vi "2400_4probesweep.vi"() -> ()   [LabVIEW 2021]
doc: "Configures a sweep and takes voltage and current readings at each point."
uses:
  <instrlib>/Keithley 24XX/Public/Data/Read (Multiple Points).vi
  <instrlib>/Keithley 24XX/Keithley 24XX.lvlib
  <vilib>/Analysis/NI_AALPro.lvlib
panel:
  out "Resistivity":dbl
  in  "Correction factor":dbl
  out "error out":errorcluster
  out "Intercept":dbl
  out "Slope":dbl
  out "XY Graph":cluster{"Current":sgl[], "Array":dbl[]}[](graph)
  in  "Source Mode  (0: Voltage)":u16(ring) items=["Voltage", "Current"]
  in  "Serial Configuration":T1={"Baud Rate"=9600, "Parity"=0, "Data Bits"=8, "Stop Bits"=10, "Flow Control"=0} {"Flow Control" items=["None", "XON/XOFF", "RTS/CTS", "XON/XOFF & RTS/CTS", "DTR/DSR", "XON/XOFF & DTR/DSR"]; "Stop Bits" items=["1.0"=10, "1.5"=15, "2.0"=20]; "Data Bits" items=["7"=7, "8"=8]; "Parity" items=["None", "Odd", "Even", "Mark", "Space"]; "Baud Rate" items=["300"=300, "600"=600, "1200"=1200, "2400"=2400, "4800"=4800, "9600"=9600, "19200"=19200]}
  in  "VISA resource name":refnum<visa-resource-name>
  out "Waveform Graph":sgl[][](graph)
  in  "Timeout (10000 ms)":i32=10000 format="%#.6g"
  in  "Maximum Amplitude (2)":dbl=2.0
  in  "Minimum Amplitude (1)":dbl=1.0
  in  "Number of Points (5)":u32=5
  in  "Compliance  Level (0.1)":dbl=0.1
  # "(c) 2006 - 2015 National Instruments.  ALL RIGHTS RESERVED."
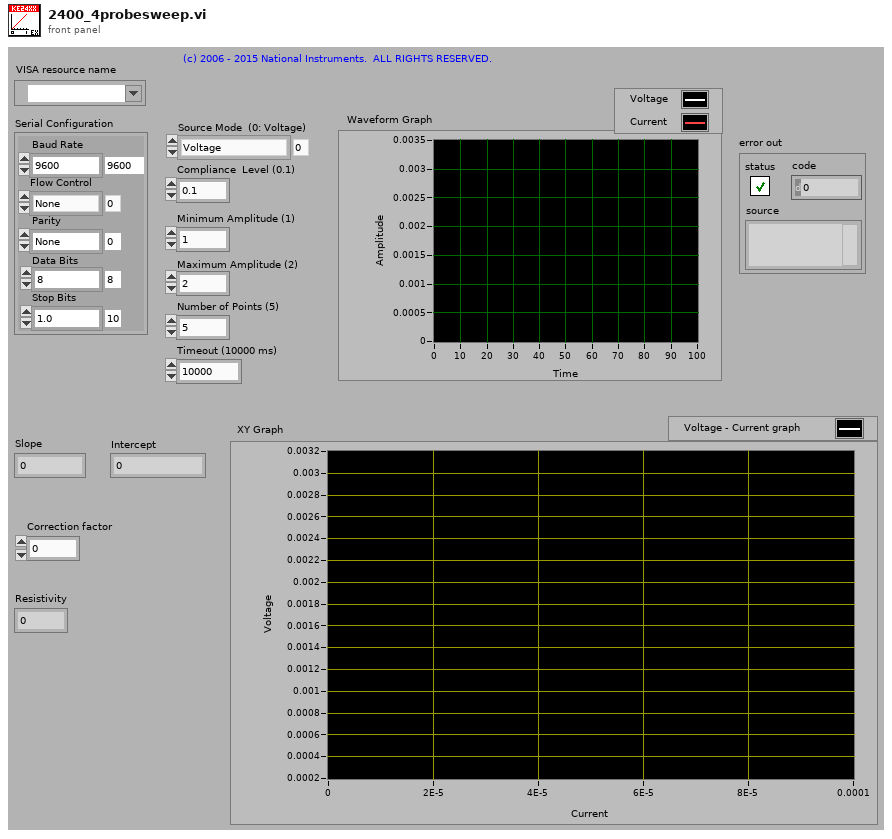
[diagram p1: front panel]
types:
  T1 = cluster{"Baud Rate":u32, "Parity":u16, "Data Bits":u16, "Stop Bits":u16, "Flow Control":u16}
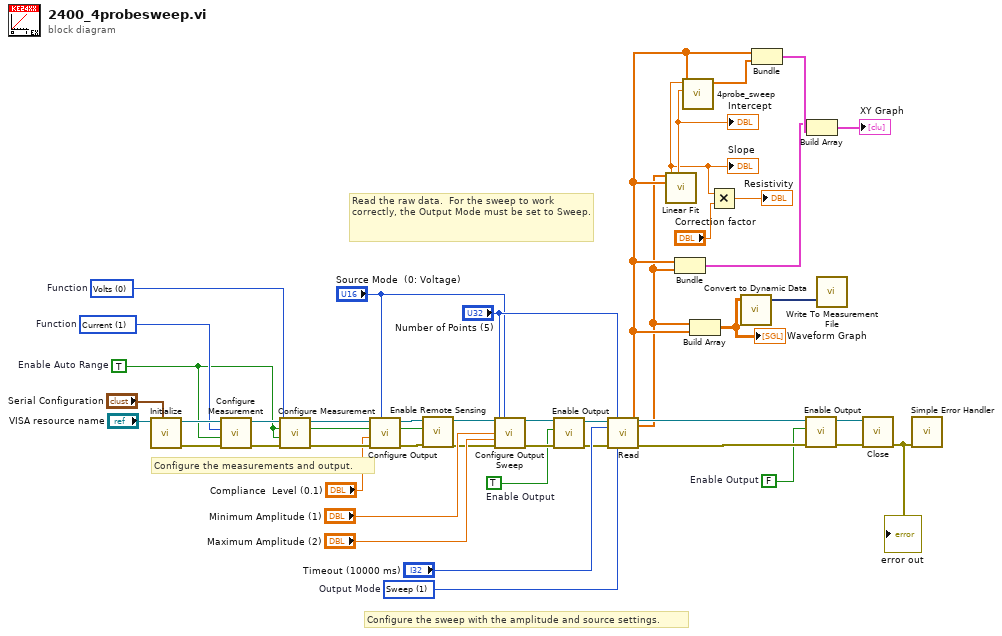
[diagram p0: block diagram]
diagram:
  w20 = TRUE  # Enable Output
  w6 = TRUE  # Enable Auto Range
  w11 = u16 0 items=["Volts", "Current", "Resistance"]  # Function
  w21 = u16 1 items=["Volts", "Current", "Resistance"]  # Function
  w27 = FALSE  # Enable Output
  w33 = u16 1 items=["Fixed", "Sweep", "List"]  # Output Mode
  # "Read the raw data.  For the sweep to work correctly, the Output Mode must be set to Sweep."
  # "Configure the sweep with the amplitude and source settings."
  # "Configure the measurements and output."
  n1 = call <instrlib>:"Initialize.vi"("Serial Configuration"="Serial Configuration", "VISA resource name"="VISA resource name") -> ("error out"=w44:errorcluster, "VISA resource name out"=w45:refnum<visa-resource-name>)  [unwired: 8 in]
  n2 = call <instrlib>:"Configure Measurement.vi"("error in (no error)"=w44, "Enable Auto Range (T:Enable)"=w6, "Function (0: Volts)"=w21, "VISA resource name"=w45) -> ("error out"=w43:errorcluster, "VISA resource name out"=w42:refnum<visa-resource-name>)  [unwired: 6 in]
  n3 = call <instrlib>:"Configure Measurement.vi"("error in (no error)"=w43, "Enable Auto Range (T:Enable)"=w6, "Function (0: Volts)"=w11, "VISA resource name"=w42) -> ("error out"=w40:errorcluster, "VISA resource name out"=w41:refnum<visa-resource-name>)  [unwired: 6 in]
  n4 = call <instrlib>:"Configure Output.vi"("Source Mode  (0: Voltage)"="Source Mode  (0: Voltage)", "error in (no error)"=w40, "Compliance  Level (0.1)"="Compliance  Level (0.1)", "VISA resource name"=w41) -> ("error out"=w8:errorcluster, "VISA resource name out"=w10:refnum<visa-resource-name>)  [unwired: 6 in]
  n5 = call <instrlib>:"Enable Remote Sensing.vi"("error in (no error)"=w8, "Enable Remote Sensing (T: Enable)"=w6, "VISA resource name"=w10) -> ("error out"=w7:errorcluster, "VISA resource name out"=w9:refnum<visa-resource-name>)  [unwired: 7 in]
  n6 = call <instrlib>:"Configure Output Sweep.vi"("VISA resource name"=w9, "Source Mode  (0: Voltage)"="Source Mode  (0: Voltage)", "Number of Points (5)"="Number of Points (5)", "Minimum Amplitude (1)"="Minimum Amplitude (1)", "Maximum Amplitude (2)"="Maximum Amplitude (2)", "error in (no error)"=w7) -> ("VISA resource name out"=w24:refnum<visa-resource-name>, "error out"=w23:errorcluster)  [unwired: 8 in]
  n7 = call <instrlib>:"Enable Output.vi"("error in (no error)"=w23, "Enable Output (T: Enable)"=w20, "VISA resource name"=w24) -> ("error out"=w26:errorcluster, "VISA resource name out"=w25:refnum<visa-resource-name>)  [unwired: 7 in]
  n8 = call-poly <instrlib>:"Read.vi"("VISA resource name"=w25, "Sample Count (1)"="Number of Points (5)", "Timeout (10000 ms)"="Timeout (10000 ms)", "error in (no error)"=w26, "Output Mode (0: Fixed)"=w33) -> ("Voltage"=w15:sgl[], "VISA resource name out"=w28:refnum<visa-resource-name>, "Current"=w16:sgl[], "error out"=w29:errorcluster)  [unwired: 4 in, 3 out]
  n9 = call <vilib>:"Linear Fit.vi"("Y"=w15, "X"=w16) -> ("slope"=w5:dbl, "intercept"=w12:dbl)  [unwired: 9 in, 3 out]
  "Slope" <- w5
  "Intercept" <- w12
  n10 = Bundle("Current"=w16, "Voltage"=w15) -> (w1:cluster{"Current":sgl[], "Voltage":sgl[]})  [unwired: 1 in]
  n11 = call "4probe_sweep.vi"("Current"=w16, "intercept"=w12, "slope"=w5) -> ("Array"=w14:dbl[])  [unwired: 8 in]
  n12 = Build Array(w15, w16) -> (w18:sgl[][])
  "Waveform Graph" <- w18
  n13 = Multiply(x=w5, y="Correction factor") -> (x*y=→"Resistivity":dbl)
  n14 = call "Convert to Dynamic Data"("2D Array"=w18) -> ("Dynamic Data Type"=w17:dynamicdata)  [unwired: 3 in]
  n15 = Bundle("Current"=w16, "Array"=w14) -> (w2:cluster{"Current":sgl[], "Array":dbl[]})  [unwired: 1 in]
  n16 = call <instrlib>:"Enable Output.vi"("error in (no error)"=w29, "Enable Output (T: Enable)"=w27, "VISA resource name"=w28) -> ("error out"=w30:errorcluster, "VISA resource name out"=w31:refnum<visa-resource-name>)  [unwired: 7 in]
  n17 = Build Array(w1, w2) -> (→"XY Graph":cluster{"Current":sgl[], "Array":dbl[]}[])
  n18 = call "Write To Measurement File"("Signals"=w17) -> ()  [unwired: 16 in, 3 out]
  n19 = call <instrlib>:"Close.vi"("error in (no error)"=w30, "VISA resource name"=w31) -> ("error out"=w32:errorcluster)  [unwired: 9 in]
  "error out" <- w32
  n20 = call <vilib>:"Simple Error Handler.vi"("error in (no error)"=w32) -> ()  [unwired: 4 in, 5 out]
